vi "Single turn magnet.vi"() -> ()   [LabVIEW 2016]
uses:
  Libraries/Utilities/Controls/Integrate channel.ctl
panel:
  out "Tektronix acquire status":string
  out "Application activity":string
  in  "Tab Control":enum32{"Fetch", "Process"}(tab)
  in  "Monitor acquire status":bool
  in  "Fetch from Tektronix":bool
  in  "Channel names to save":string[](array[string])=["Trig init", "Trig delay", "BdotSafe", "Bdot"]
  in  "Fetch channels":u16[](array[ring])=[0, 1, 2, 3] items=["Channel 1", "Channel 2", "Channel 3", "Channel 4", "Math", "Reference 1", "Reference 2", "Reference 3", "Reference 4", "D0", "D1", "D2", "D3", "D4", "D5", "D6", "D7", "D8", "D9", "D10", "D11", "D12", "D13", "D14", "D15", "Amplitude", "Frequency", "Phase", "Normal", "Average", "Maximum Peak Hold", "Minimum Peak Hold"]
  out "Tektronix data":waveform(dbl)[](graph)
  in  "VISA resource name":refnum<visa-resource-name>="USB0::0x0699::0x0401::C011905::INSTR"
  in  "Export to ASCII":bool
  in  "Attenuation":dbl=100.0
  in  "terminator W":dbl
  in  "coil W":dbl
  in  "Comments":string="Pulse info:"
  in  "Export":bool
  in  "Offset correction":dbl
  in  "Integrate Button":bool
  out "Min max result":cluster{"Max":dbl, "Min":dbl}
  out "Waveform Graph":waveform(dbl)(graph)
  in  "Integration settings":T1={"Channel"="Bdot", "Output name"="Field", "Factor"=1350000.0, "Start time"=0.0, "Duration"=0.0, "Fix drift"=FALSE} {"Duration" format="%#_6ps"; "Start time" format="%#_6ps"}
  in  "Offset duration":dbl=1e-05
  in  "TDMS File Path":path
  out "dt":dbl format="%#_6p"
  in  "Stop Button":bool
  # "...to TDMS file"
  # "Bdot name  -  Factor   - Output name"
  # "s"
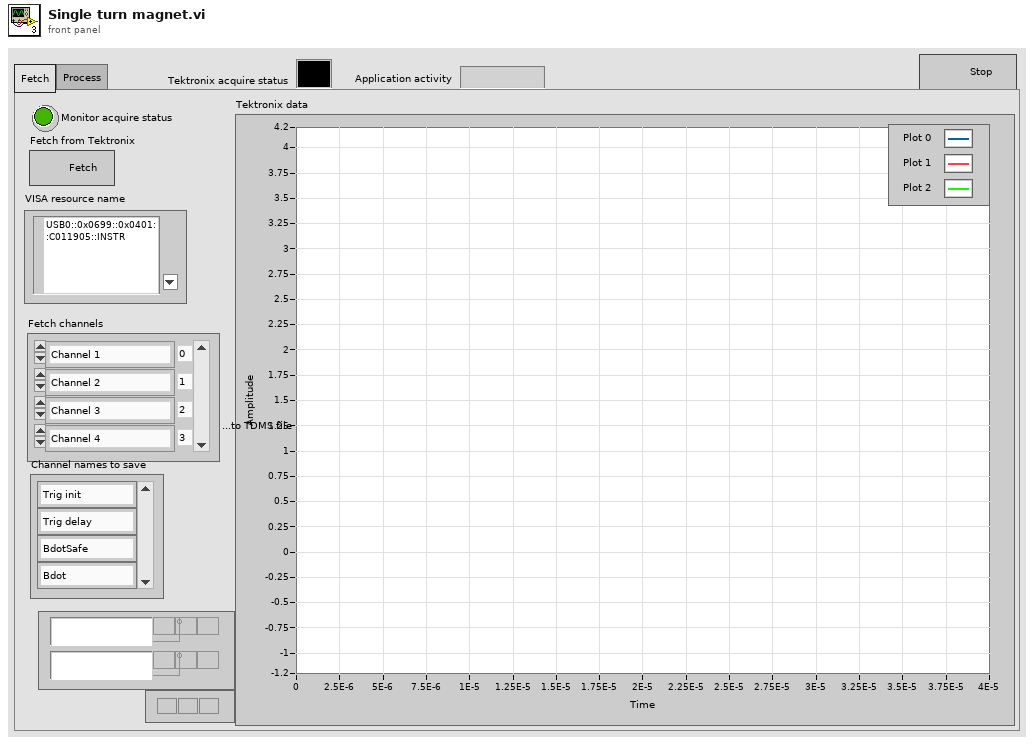
[diagram p1: front panel]
types:
  T1 = typedef "Integrate channel.ctl" = cluster{"Channel":string, "Output name":string, "Factor":dbl, "Start time":dbl, "Duration":dbl, "Fix drift":bool}
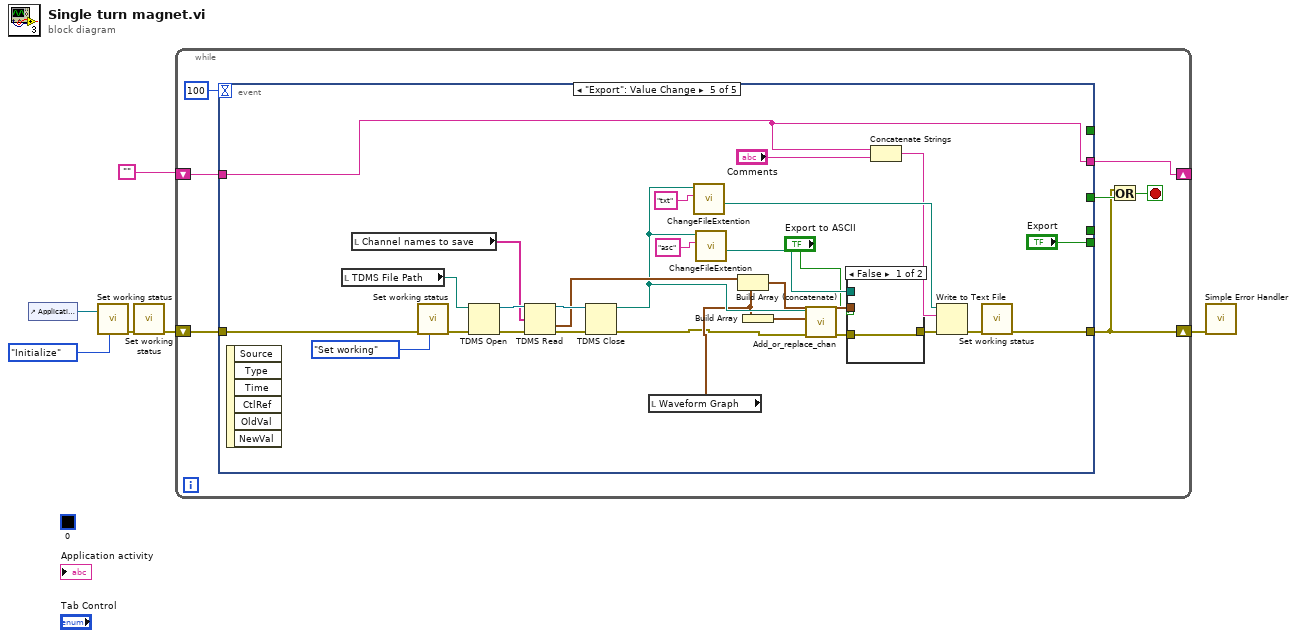
[diagram p0: block diagram]
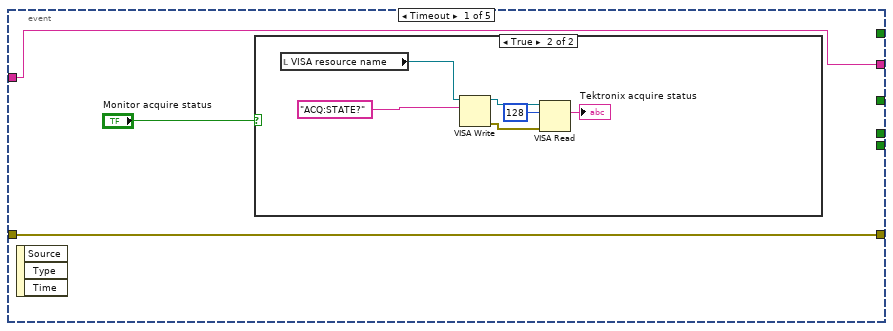
[diagram p2: hidden frame]
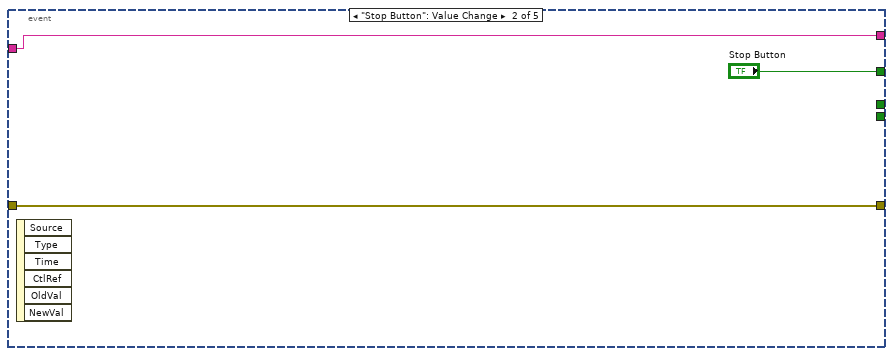
[diagram p4: hidden frame]
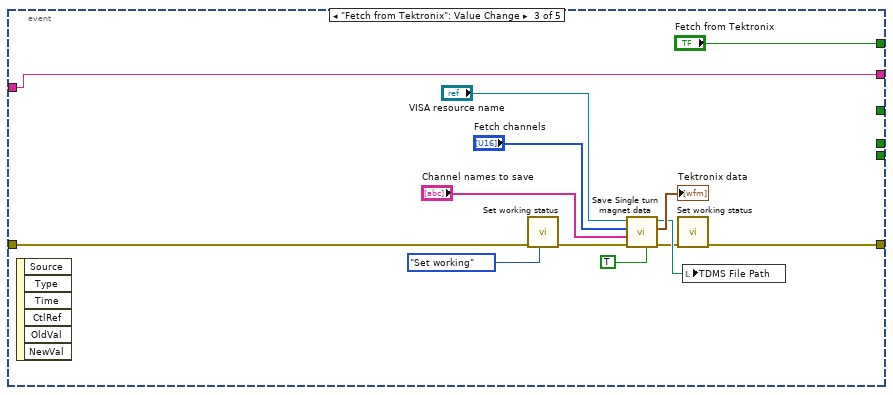
[diagram p5: hidden frame]
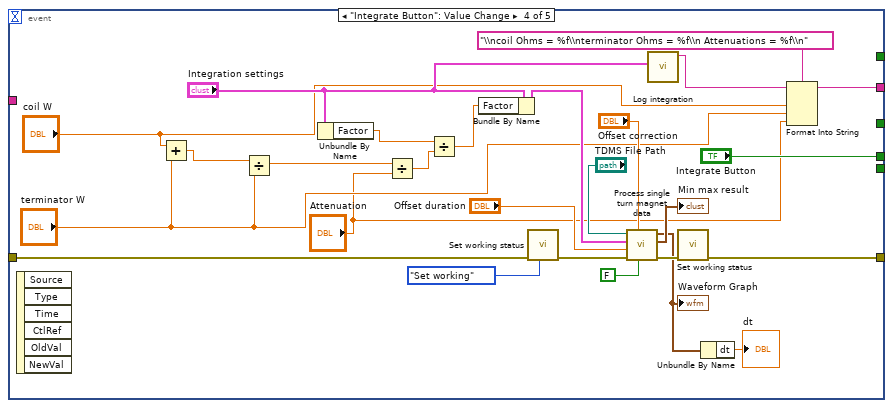
[diagram p6: hidden frame]
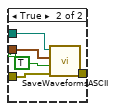
[diagram p7: hidden frame]
diagram:
  (unwired) u32 0
  n1 = control-ref of="Application activity"() -> (w5:refnum<vi>)
  n2 = call "Set working status.vi"("Enum"=enum16{"Set done", "Set working", "Initialize"}."Initialize", "reference"=w5) -> ("Error Out"=w3:errorcluster)  [unwired: 9 in]
  n3 = call "Set working status.vi"("Error In"=w3) -> ("Error Out"=w2:errorcluster)  [unwired: 10 in]
  n4 = while {
    shift-right: [w10] -> w6
    shift-left: w2 -> [w12]
    shift-right: [w7] -> _
    shift-left: "" -> [w8]
    stop <- w11 stop-if-true
    n5 = event shown="[4] \"Export\": Value Change" {
      selector: _ -> [_ _ _ _ _]
      dyn-events: _ -> [_ _ _ _ _]
      timeout: 100 -> [_ _ _ _ _]
      tunnel: [_ "Stop Button" _ _ _] -> w13
      tunnel: [_ _ "Fetch from Tektronix" _ _] -> _
      tunnel: [w16 w24 w27 w54 w81] -> w10
      tunnel: w12 -> [w16 w24 w31 w58 w80]
      tunnel: [_ _ _ "Integrate Button" _] -> _
      tunnel: [_ _ _ _ "Export"] -> _
      tunnel: w8 -> [w14 w23 w26 _ w69]
      tunnel: [w14 w23 w26 w41 w69] -> w7
      event Timeout {
        n6 = event-data() -> ()  [unwired: 1 in, 3 out]
        n7 = case shown="True" "Monitor acquire status" {
          frame False {
          }
          frame True {
            n8 = local read "VISA resource name"() -> (w17:refnum<visa-resource-name>)
            n9 = VISA Write(VISA resource name=w17, write buffer="ACQ:STATE?") -> (VISA resource name out=w21:refnum<visa-resource-name>, error out=w19:errorcluster)  [unwired: 1 in, 1 out]
            n10 = VISA Read(VISA resource name=w21, byte count=u32 128, error in (no error)=w19) -> (read buffer=→"Tektronix acquire status":string)  [unwired: 3 out]
          }
        }
      }
      event "Stop Button": Value Change {
        n11 = event-data() -> ()  [unwired: 1 in, 6 out]
      }
      event "Fetch from Tektronix": Value Change {
        n12 = event-data() -> ()  [unwired: 1 in, 6 out]
        n13 = call "Set working status.vi"("Enum"=enum16{"Set done", "Set working", "Initialize"}."Set working", "Error In"=w31) -> ("Error Out"=w30:errorcluster)  [unwired: 9 in]
        n14 = call "Save Single turn magnet data.vi"("Save data"=TRUE, "Error In"=w30, "Channel names to save"="Channel names to save", "Fetch channels"="Fetch channels", "VISA resource name"="VISA resource name") -> ("Error Out"=w28:errorcluster, "Waveform Graph"=→"Tektronix data":waveform(dbl)[], "File Path"=w33:path)  [unwired: 4 in]
        n15 = call "Set working status.vi"("Error In"=w28) -> ("Error Out"=w27:errorcluster)  [unwired: 10 in]
        n16 = local write "TDMS File Path"(w33) -> ()
      }
      event "Integrate Button": Value Change {
        n17 = event-data() -> ()  [unwired: 1 in, 6 out]
        n18 = Add(x="coil W", y="terminator W") -> (x+y=w50:dbl)
        n19 = Divide(x=w50, y="terminator W") -> (x/y=w51:dbl)
        n20 = Unbundle By Name("Integration settings") -> ("Factor"=w49:dbl)
        n21 = Divide(x=w51, y="Attenuation") -> (x/y=w48:dbl)
        n22 = Divide(x=w49, y=w48) -> (x/y=w46:dbl)
        n23 = Bundle By Name(cluster="Integration settings", "Factor"=w46) -> (w47:T1)
        n24 = call "Set working status.vi"("Enum"=enum16{"Set done", "Set working", "Initialize"}."Set working", "Error In"=w58) -> ("Error Out"=w57:errorcluster)  [unwired: 9 in]
        n25 = call "Process single turn magnet data.vi"("Save data"=FALSE, "Offset correction"="Offset correction", "Error In"=w57, "Offset duration"="Offset duration", "Integration settings"=w47, "File Path Control"="TDMS File Path") -> ("Error Out"=w55:errorcluster, "Min max"=→"Min max result":cluster{"Max":dbl, "Min":dbl}, "Waveform Graph"=w53:waveform(dbl))  [unwired: 3 in]
        "Waveform Graph" <- w53
        n26 = call "Log integration.vi"("Integration settings"="Integration settings") -> ("String out"=w44:string)  [unwired: 7 in, 3 out]
        n27 = call "Set working status.vi"("Error In"=w55) -> ("Error Out"=w54:errorcluster)  [unwired: 10 in]
        n28 = Unbundle By Name(w53) -> ("dt"=→"dt":dbl)
        n29 = Format Into String(format string="\\ncoil Ohms = %f\\nterminator Ohms = %f\\n Attenuations = %f\\n", initial string=w44, "coil W", "terminator W", "Attenuation") -> (resulting string=w41:string)  [unwired: 1 in, 1 out]
      }
      event "Export": Value Change {
        n30 = event-data() -> ()  [unwired: 1 in, 6 out]
        n31 = local read "TDMS File Path"() -> (w86:path)
        n32 = local read "Channel names to save"() -> (w84:string[])
        n33 = call "Set working status.vi"("Enum"=enum16{"Set done", "Set working", "Initialize"}."Set working", "Error In"=w80) -> ("Error Out"=w79:errorcluster)  [unwired: 9 in]
        n34 = TDMS Open(8:w79, 11:w86) -> (0:w85:errorcluster, 3:w87:refnum<k34>)  [unwired: 5 in]
        n35 = TDMS Read(0:w87, 7:w84, 11:w85) -> (4:w88:refnum<k34>, 10:w83:waveform(dbl)[], 15:w89:errorcluster)  [unwired: 5 in, 3 out]
        n36 = TDMS Close(8:w89, 11:w88) -> (0:w66:errorcluster, 3:w71:path)
        n37 = local read "Waveform Graph"() -> (w67:waveform(dbl))
        n38 = call "ChangeFileExtention.vi"("New extension"="txt" ("New Extention"), "File Path"=w71) -> ("Path with new extension"=w73:path)  [unwired: 4 in, 5 out]
        n39 = call "ChangeFileExtention.vi"("New extension"="asc" ("New Extention"), "File Path"=w71) -> ("Path with new extension"=w90:path)  [unwired: 4 in, 5 out]
        n40 = Build Array (concatenate)(w83, w67) -> (w82:waveform(dbl)[])
        n41 = Build Array(w67) -> (w68:waveform(dbl)[])
        n42 = call "Add_or_replace_chan.vi"("Error In"=w66, "Waveforms"=w68, "File Path Control"=w71) -> ("Error Out"=w72:errorcluster)  [unwired: 5 in, 3 out]
        n43 = case shown="False" "Export to ASCII" {
          tunnel: w90 -> [_ w98]
          tunnel: w82 -> [_ w97]
          tunnel: [w93 w95] -> w76
          tunnel: w72 -> [w93 w94]
          frame False {
          }
          frame True {
            n44 = call "SaveWaveformsASCII.vi"("Error In"=w94, "Save column names"=TRUE, "Waveforms"=w97, "File"=w98) -> ("Error Out"=w95:errorcluster)  [unwired: 6 in, 1 out]
          }
        }
        n45 = Concatenate Strings(w69, "Comments") -> (w70:string)
        n46 = Write to Text File(file (use dialog)=w73, text=w70, error in=w76) -> (error out=w75:errorcluster)  [unwired: 1 in, 2 out]
        n47 = call "Set working status.vi"("Error In"=w75) -> ("Error Out"=w81:errorcluster)  [unwired: 10 in]
      }
    }
    n48 = Or(x=w10, y=w13) -> (x .or. y?=w11:bool)
  }
  n49 = call <vilib>:"Simple Error Handler.vi"("error in (no error)"=w6) -> ()  [unwired: 4 in, 5 out]
